vi "worker_loop.vi"(8 "error in (no error)":errorcluster, 10 "Notifiers":T1, 11 "Message Queues":T2) -> (0 "error out":errorcluster)   [LabVIEW 2017, in "worker.lvlib"]
uses:
  worker.lvlib
  support/Message Queue/All Message Queues.ctl
  support/Message Queue/Message Cluster.ctl
  support/Notifiers/Notifiers.ctl
  support/my_global.vi
  <vilib>/Utility/error.llb/Error Cluster From Error Code.vi
  <vilib>/ErrorRing/Error Ring.xnode
  support/Message Queue/Message Queue.lvlib
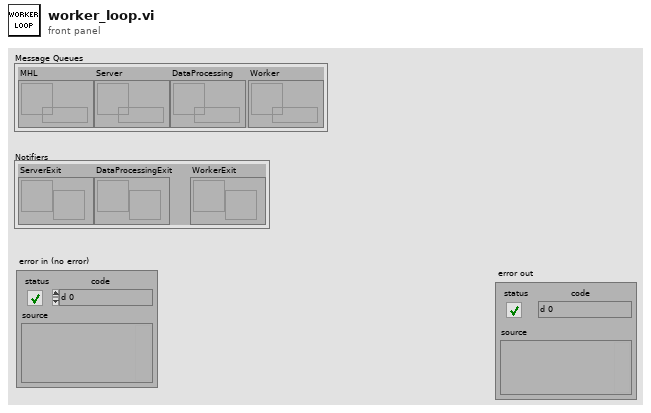
[diagram p1: front panel]
types:
  T1 = typedef "Notifiers.ctl" = cluster{"ServerExit":refnum<notifier>, "DataProcessingExit":refnum<notifier>, "WorkerExit":refnum<notifier>}
  T2 = typedef "Message Queue.lvlib/All Message Queues.ctl" = cluster{"MHL":refnum<queue>, "Server":refnum<queue>, "DataProcessing":refnum<queue>, "Worker":refnum<queue>}
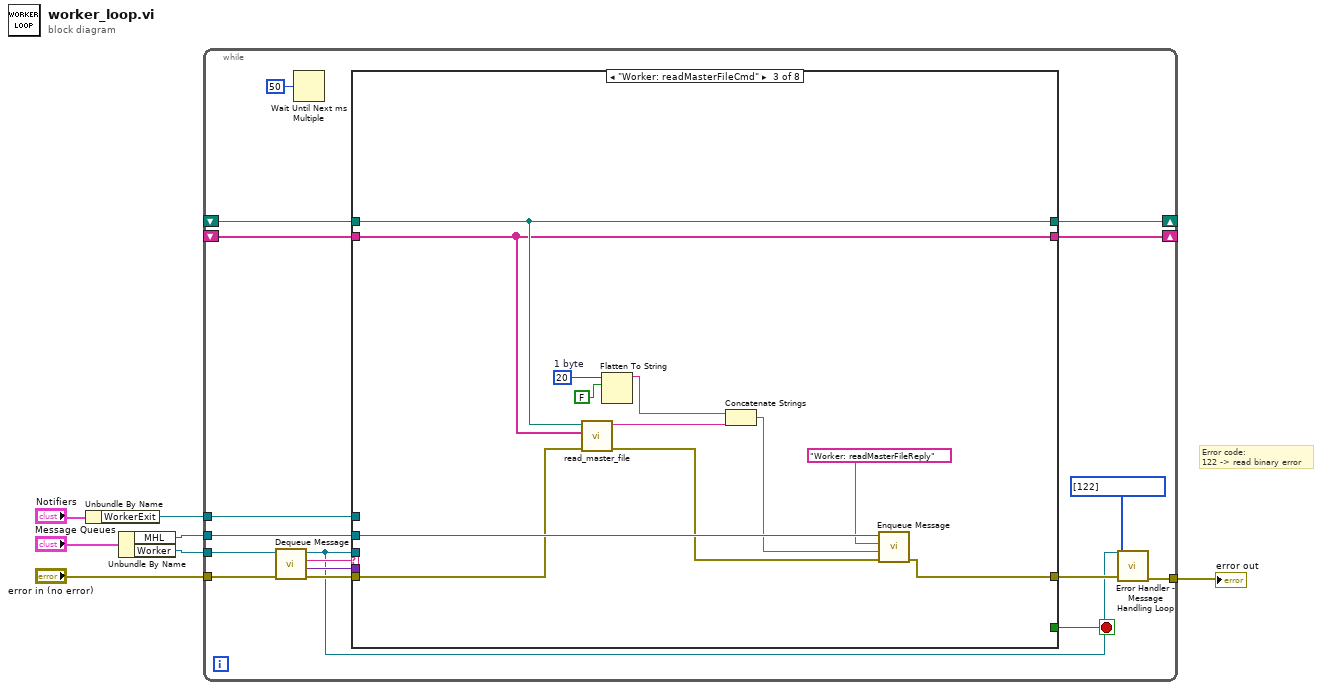
[diagram p0: block diagram]
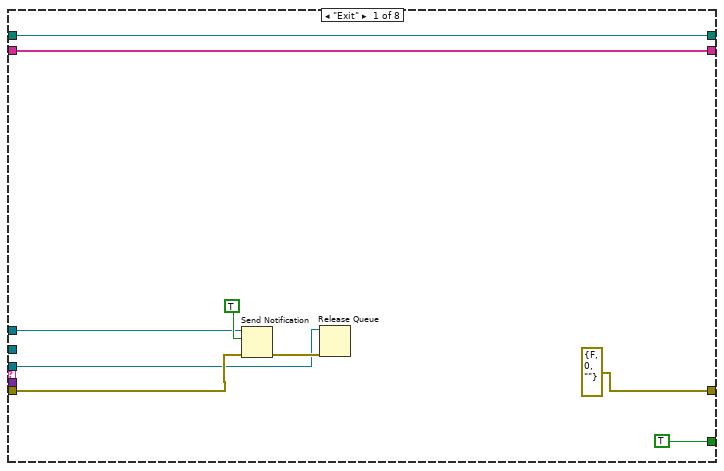
[diagram p2: hidden frame]
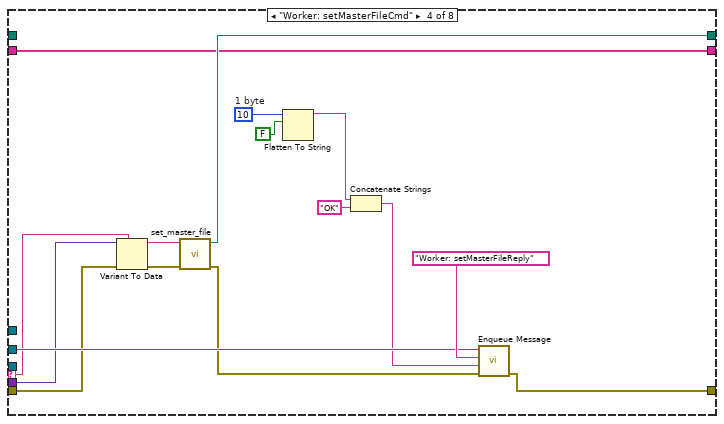
[diagram p4: hidden frame]
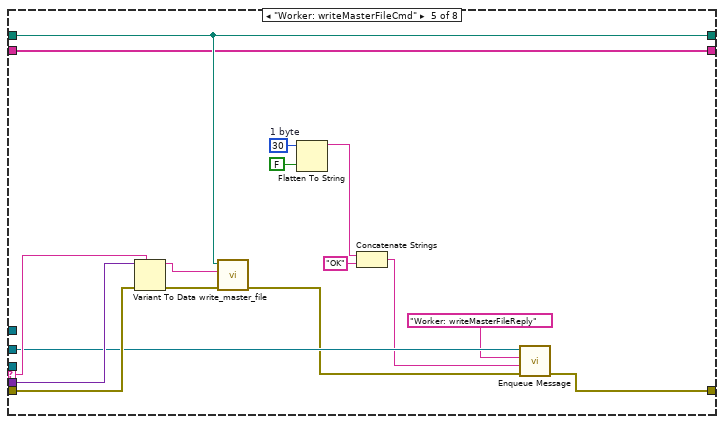
[diagram p5: hidden frame]
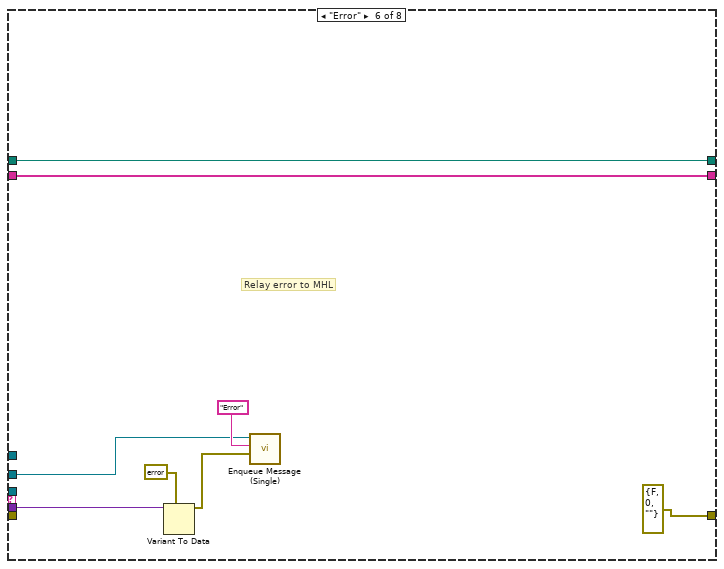
[diagram p6: hidden frame]
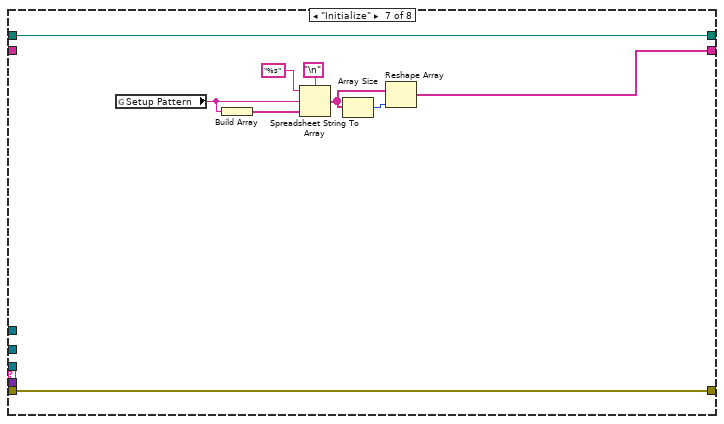
[diagram p7: hidden frame]
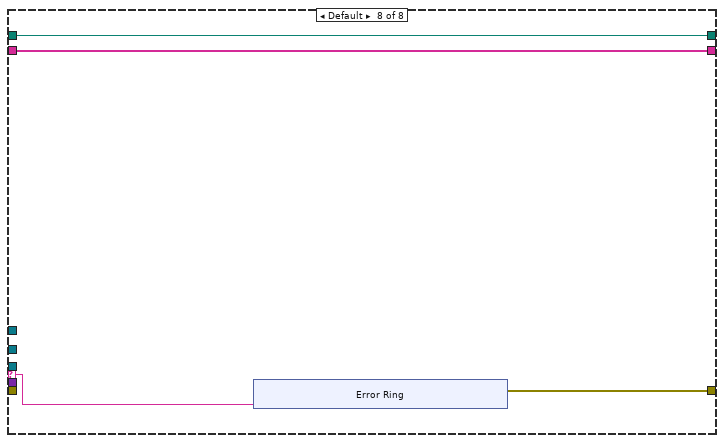
[diagram p8: hidden frame]
diagram:
  # "Error code:\n122 -> read binary error"
  n1 = Unbundle By Name("Notifiers") -> ("WorkerExit"=w3:refnum<notifier>)
  n2 = Unbundle By Name("Message Queues") -> ("MHL"=w6:refnum<queue>, "Worker"=w5:refnum<queue>)
  n3 = while {
    tunnel: w6 -> [w18]
    tunnel: w5 -> [w23]
    tunnel: w3 -> [w13]
    tunnel: "error in (no error)" -> [w22]
    tunnel: [w15] -> w1
    shift-right: [w12] -> _
    shift-left: _ -> [w11]
    shift-right: [w10] -> _
    shift-left: _ -> [w9]
    stop <- w14 stop-if-true
    n4 = call "Dequeue Message.vi"("error in (no error)"=w22, "Message Queue"=w23) -> ("error out"=w19:errorcluster, "Message Data"=w20:variant, "Message"=w21:string, "dup Message Queue"=w16:refnum<queue>)  [unwired: 6 in]
    n5 = Wait Until Next ms Multiple(millisecond multiple=u32 50) -> ()  [unwired: 1 out]
    n6 = case shown="\"Worker: readMasterFileCmd\"" w21 {
      selector: w21 -> [_ _ _ w57 w79 _ _ w101]
      tunnel: w16 -> [w29 _ _ _ _ _ _ _]
      tunnel: w20 -> [_ _ _ w56 w80 w84 _ _]
      tunnel: w19 -> [w30 w36 w39 w55 w78 _ w97 _]
      tunnel: w18 -> [_ _ w48 w62 w76 w83 _ _]
      tunnel: [errorcluster {"status"=FALSE, "code"=0, "source"=""} ("error constant") w36 w47 w63 w77 errorcluster {"status"=FALSE, "code"=0, "source"=""} ("error constant") w97 w100] -> w17
      tunnel: [TRUE _ _ _ _ _ _ _] -> w14
      tunnel: w13 -> [w28 _ _ _ _ _ _ _]
      tunnel: [w26 w35 w38 w50 w67 w82 w96 w99] -> w12
      tunnel: w11 -> [w26 w35 w38 _ w67 w82 w96 w99]
      tunnel: [w25 w34 w37 w49 w66 w81 w89 w98] -> w10
      tunnel: w9 -> [w25 w34 w37 w49 w66 w81 _ w98]
      frame "Exit" {
        n7 = Send Notification(notification=TRUE, notifier=w28, error in (no error)=w30) -> (error out=w31:errorcluster)  [unwired: 1 out]
        n8 = Release Queue(queue=w29, error in (no error)=w31) -> ()  [unwired: 1 in, 3 out]
      }
      frame "--- Copy me ---" {
      }
      frame "Worker: readMasterFileCmd" {
        w45 = u8 20  # 1 byte
        n9 = call "read_master_file.vi"("error in (no error)"=w39, "setup file pattern"=w37, "master file path"=w38) -> ("error out"=w43:errorcluster, "setup file paths"=w42:string)  [unwired: 7 in]
        n10 = Flatten To String(anything=w45, prepend array or string size? (T)=FALSE) -> (data string=w41:string)  [unwired: 2 in, 2 out]
        n11 = Concatenate Strings(w41, w42) -> (w40:string)
        n12 = call-poly "Enqueue Message.vi"("error in (no error)"=w43, "Message Data"=w40, "Message"="Worker: readMasterFileReply", "Message Queue"=w48) -> ("error out"=w47:errorcluster)  [unwired: 6 in, 1 out]
      }
      frame "Worker: setMasterFileCmd" {
        w61 = u8 10  # 1 byte
        n13 = Variant To Data(error in=w55, type=w57, Variant=w56) -> (data=w53:string, error out=w54:errorcluster)
        n14 = call "set_master_file.vi"("error in (no error)"=w54, "master file path"=w53) -> ("error out"=w51:errorcluster, "master file path"=w50:path)  [unwired: 8 in]
        n15 = Flatten To String(anything=w61, prepend array or string size? (T)=FALSE) -> (data string=w59:string)  [unwired: 2 in, 2 out]
        n16 = Concatenate Strings(w59, "OK" ("string")) -> (w58:string)
        n17 = call-poly "Enqueue Message.vi"("error in (no error)"=w51, "Message Data"=w58, "Message"="Worker: setMasterFileReply", "Message Queue"=w62) -> ("error out"=w63:errorcluster)  [unwired: 6 in, 1 out]
      }
      frame "Worker: writeMasterFileCmd" {
        w73 = u8 30  # 1 byte
        n18 = Variant To Data(error in=w78, type=w79, Variant=w80) -> (data=w65:string, error out=w75:errorcluster)
        n19 = call "write_master_file.vi"("error in (no error)"=w75, "setup file paths"=w65, "master file path"=w67) -> ("error out"=w74:errorcluster)  [unwired: 8 in]
        n20 = Flatten To String(anything=w73, prepend array or string size? (T)=FALSE) -> (data string=w71:string)  [unwired: 2 in, 2 out]
        n21 = Concatenate Strings(w71, "OK" ("string")) -> (w70:string)
        n22 = call-poly "Enqueue Message.vi"("error in (no error)"=w74, "Message Data"=w70, "Message"="Worker: writeMasterFileReply", "Message Queue"=w76) -> ("error out"=w77:errorcluster)  [unwired: 6 in, 1 out]
      }
      frame "Error" {
        # "Relay error to MHL"
        n23 = Variant To Data(type=errorcluster {"status"=FALSE, "code"=0, "source"=""} ("error constant"), Variant=w84) -> (data=w86:errorcluster)  [unwired: 1 in, 1 out]
        n24 = call "Enqueue Message (Single).vi"("Message Data"=w86, "Message"="Error", "Message Queue"=w83) -> ()  [unwired: 7 in, 2 out]
      }
      frame "Initialize" {
        n25 = global read "my_global.vi" "Setup Pattern"() -> (w95:string)
        n26 = Build Array(w95) -> (w94:string[])
        n27 = Spreadsheet String To Array(delimiter (Tab)="\n", format string="%s", spreadsheet string=w95, array type (2D Dbl)=w94) -> (array=w90:string[])
        n28 = Array Size(array=w90) -> (size(s)=w93:i32)
        n29 = Reshape Array(w90, w93) -> (w89:string[])
      }
      frame Default {
        n30 = xnode "Error Ring"("parameter 0"=w101) -> ("error out"=w100:errorcluster)
      }
    }
    n31 = call "Error Handler - Message Handling Loop.vi"("error in (no error)"=w17, "Ignore Errors (Runtime)"=i32[] [122], "Message Queue"=w16) -> ("dup error in"=w15:errorcluster)  [unwired: 7 in, 1 out]
  }
  "error out" <- w1
